vi "LoggingOperation.vi"(8 "Operation":T1, 10 "Data":variant, 11 "Name":string) -> (3 "Log String":string)   [LabVIEW 2017]
uses:
  LogOperation.ctl
  <vilib>/Utility/Data Type/NI_Data Type.lvlib
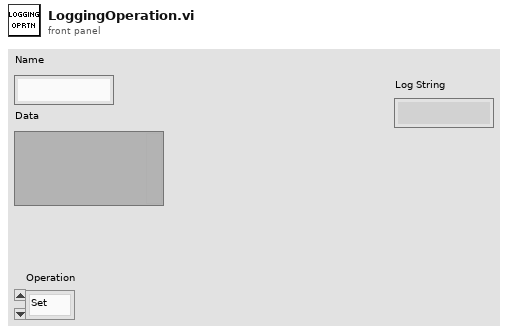
[diagram p1: front panel]
types:
  T1 = typedef "LogOperation.ctl" = enum16{"Set", "Get All", "Init"}
  T2 = typedef "NI_Data Type.lvlib/Data Type.ctl" = enum8{"Invalid Type", "Void", "I8", "I16", "I32", "I64", "U8", "U16", "U32", "U64", "Single Float", "Double Float", "Extended Float", "Single Complex", "Double Complex", "Extended Complex", "Enum U8", "Enum U16", "Enum U32", "Enum U64", "Single Float With Unit", "Double Float With Unit", "Extended Float With Unit", "Single Complex with Unit", "Double Complex with Unit", "Extended Complex with Unit", "Boolean", "String", "Path", "Picture", "Tag", "Array", "Cluster", "Variant", "LV Variant", "Waveform", "Timestamp", "Digital Waveform", "Digital Data", "ExpressData", "Refnum", "External Data", "VI", "Poly VI", "LabVIEW Class Instance", "Fixed Point"}
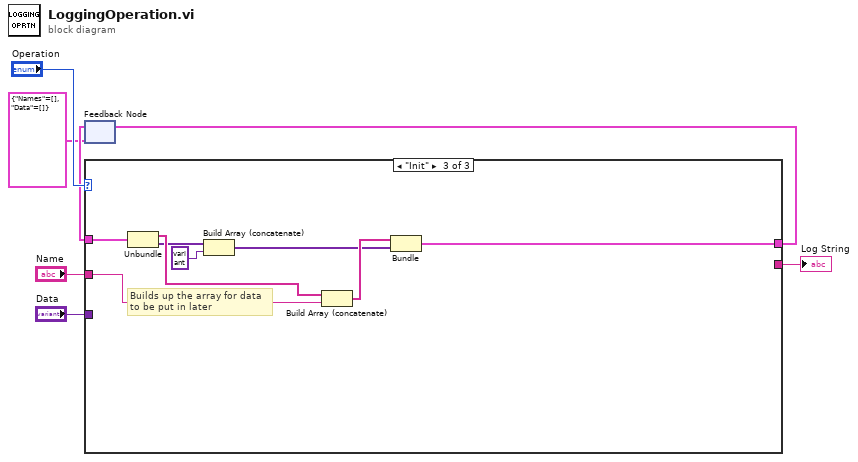
[diagram p0: block diagram]
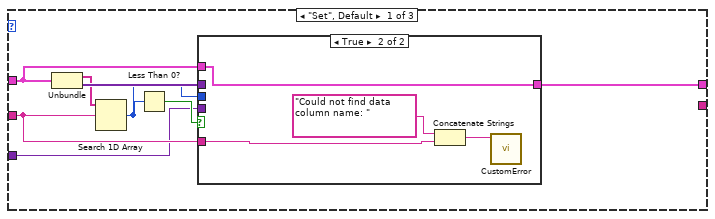
[diagram p2: hidden frame]
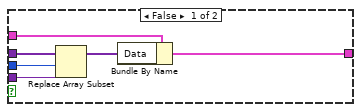
[diagram p3: hidden frame]
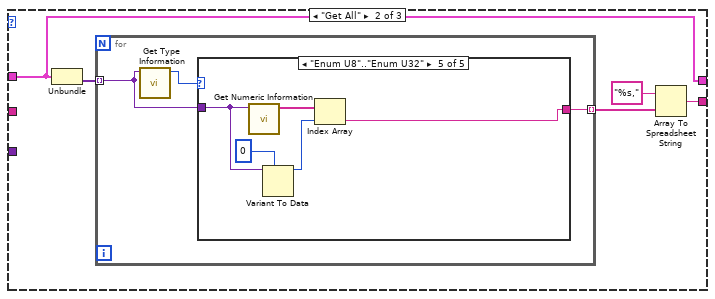
[diagram p4: hidden frame]
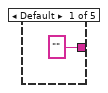
[diagram p5: hidden frame]
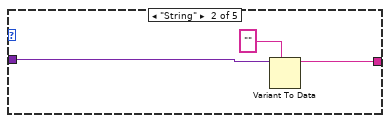
[diagram p6: hidden frame]
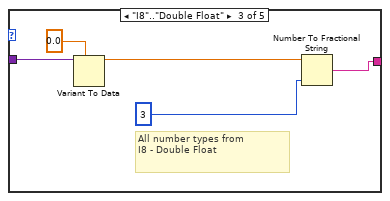
[diagram p7: hidden frame]
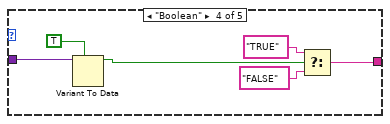
[diagram p8: hidden frame]
diagram:
  n1 = feedback #1(cluster{"Names":string[], "Data":variant[]} {"Names"=[], "Data"=[]}) -> (w6:cluster{"Names":string[], "Data":variant[]})
  n2 = case shown="\"Init\"" "Operation" {
    tunnel: w6 -> [w8 w30 w61]
    tunnel: [w9 w30 w54] -> w3
    tunnel: "Name" -> [w14 _ w57]
    tunnel: "Data" -> [w11 _ _]
    tunnel: [_ w27 _] -> w1
    frame "Set", Default {
      n3 = Unbundle(w8) -> ("Names"=w10:string[], "Data"=w13:variant[])
      n4 = Search 1D Array(1D array=w10, element=w14) -> (index of element=w12:i32)  [unwired: 1 in]
      n5 = Less Than 0?(x=w12) -> (x < 0?=w15:bool)
      n6 = case shown="True" w15 {
        tunnel: w14 -> [_ w23]
        tunnel: w13 -> [w21 _]
        tunnel: w12 -> [w20 _]
        tunnel: w11 -> [w19 _]
        tunnel: [w16 w22] -> w9
        tunnel: w8 -> [w18 w22]
        frame False {
          n7 = Replace Array Subset(array=w21, new element=w19, index=w20) -> (w17:variant[])
          n8 = Bundle By Name(cluster=w18, "Data"=w17) -> (w16:cluster{"Names":string[], "Data":variant[]})
        }
        frame True {
          n9 = Concatenate Strings("Could not find data column name: ", w23) -> (w24:string)
          n10 = call "CustomError.vi"("String"=w24) -> ()  [unwired: 10 in, 1 out]
        }
      }
    }
    frame "Get All" {
      n11 = Unbundle(w30) -> ("Data"=w29:variant[])  [unwired: 1 out]
      n12 = for {
        tunnel: w29 -> [w32] mode=indexing
        tunnel: [w33] -> w26 mode=indexing
        n13 = call <vilib>:"Get Type Information.vi"("Variant"=w32) -> ("Type"=w31:T2)  [unwired: 6 in, 4 out]
        n14 = case shown="\"Enum U8\"..\"Enum U32\"" w31 {
          tunnel: ["" ("Name") w36 w38 w43 w49] -> w33
          tunnel: w32 -> [_ w37 w42 w48 w50]
          frame Default {
          }
          frame "String" {
            n15 = Variant To Data(type="" ("Name"), Variant=w37) -> (data=w36:string)  [unwired: 1 in, 1 out]
          }
          frame "I8".."Double Float" {
            # "All number types from\nI8 - Double Float"
            n16 = Variant To Data(type=0.0, Variant=w42) -> (data=w40:dbl)  [unwired: 1 in, 1 out]
            n17 = Number To Fractional String(number=w40, precision (6)=i16 3) -> (F-format string=w38:string)  [unwired: 2 in]
          }
          frame "Boolean" {
            n18 = Variant To Data(type=TRUE, Variant=w48) -> (data=w46:bool)  [unwired: 1 in, 1 out]
            n19 = Select(t="TRUE" ("format string"), s=w46, f="FALSE" ("format string")) -> (s? t:f=w43:string)
          }
          frame "Enum U8".."Enum U32" {
            n20 = call <vilib>:"Get Numeric Information.vi"("Variant"=w50) -> ("Enum Names"=w53:string[])  [unwired: 7 in, 3 out]
            n21 = Variant To Data(type=u32 0 ("milliseconds to wait"), Variant=w50) -> (data=w51:u32)  [unwired: 1 in, 1 out]
            n22 = Index Array(array=w53, index=w51) -> (element=w49:string)
          }
        }
      }
      n23 = Array To Spreadsheet String(array=w26, 3:"%s," ("format string")) -> (spreadsheet string=w27:string)  [unwired: 1 in]
    }
    frame "Init" {
      # "Builds up the array for data\nto be put in later"
      n24 = Unbundle(w61) -> ("Names"=w60:string[], "Data"=w59:variant[])
      n25 = Build Array (concatenate)(w59, variant ("Data")) -> (w55:variant[])
      n26 = Build Array (concatenate)(w60, w57) -> (w56:string[])
      n27 = Bundle(w56, w55) -> (w54:cluster{string[], variant[]})  [unwired: 1 in]
    }
  }
  "Log String" <- w1
  n28 = feedback-in #1(w3) -> ()
